vi "Frame Sync.vi"(6 "channel count (2)":u8=2, 7 "bit set edge (falling)":enum16{"rising", "falling"}(ring)=enum."falling", 9 "ready for input?":bool, 10 "transmit":bool, 11 "clock in":bool) -> (1 "ready for input":bool, 2 "latch config":bool, 3 "frame sync":bool)   [LabVIEW 2013, in "I2S-TDM.lvlib"]
uses:
  I2S-TDM.lvlib
  Controls/tdm transmit states.ctl
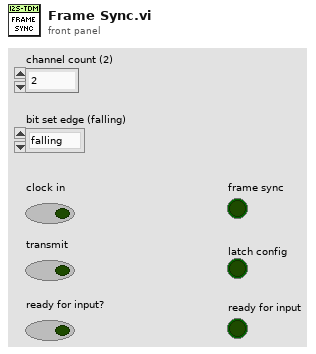
[diagram p1: front panel]
types:
  T1 = typedef "I2S-TDM.lvlib/tdm transmit states.ctl" = enum16{"idle", "pre-transfer", "transfer"}
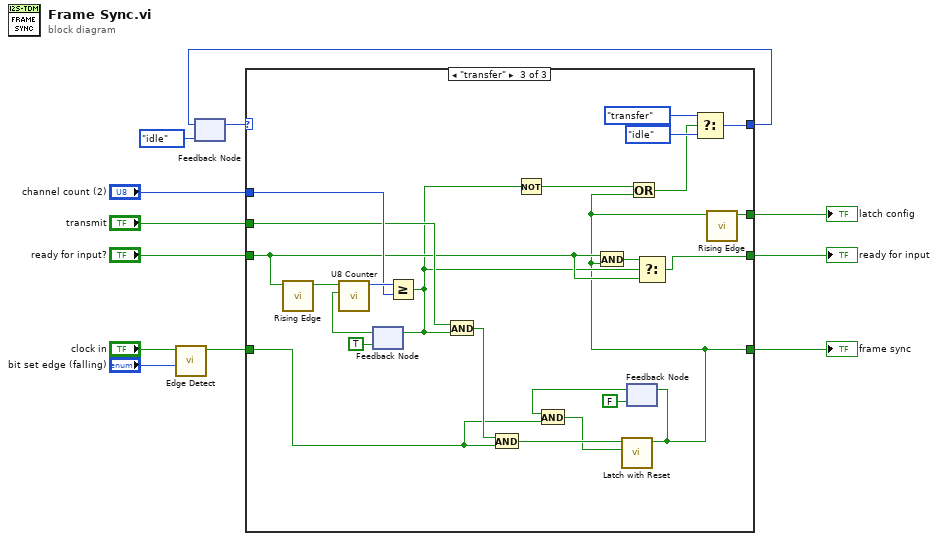
[diagram p0: block diagram]
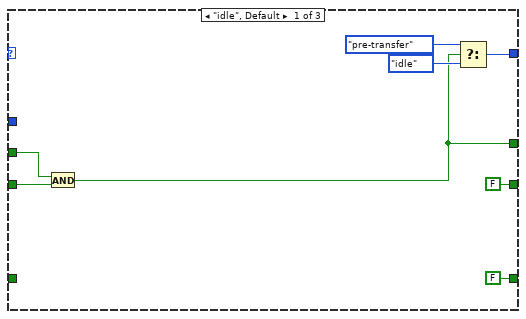
[diagram p2: hidden frame]
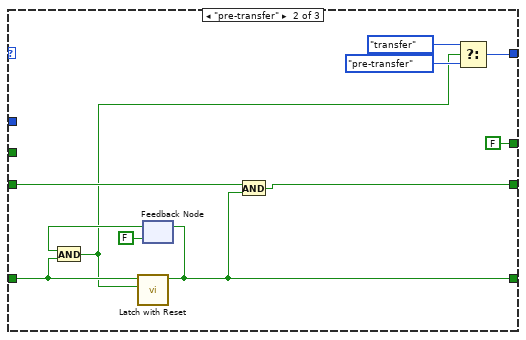
[diagram p3: hidden frame]
diagram:
  n1 = call "Edge Detect.vi"("edge (rising)"="bit set edge (falling)", "signal in"="clock in") -> ("edge detected?"=w6:bool)  [unwired: 9 in]
  n2 = feedback #1(tdm_transmit_states."idle") -> (w11:T1)
  n3 = case shown="\"transfer\"" w11 {
    tunnel: [w16 w26 w52] -> w10
    tunnel: "transmit" -> [w19 _ w48]
    tunnel: "ready for input?" -> [w20 w30 w42]
    tunnel: w6 -> [_ w25 w40]
    tunnel: [FALSE w29 w43] -> w5
    tunnel: [FALSE ("latched signal") w22 w32] -> w4
    tunnel: "channel count (2)" -> [_ _ w49]
    tunnel: [w13 FALSE w34] -> w2
    frame "idle", Default {
      n4 = And(x=w19, y=w20) -> (x .and. y?=w13:bool)
      n5 = Select(t=tdm_transmit_states."pre-transfer", s=w13, f=tdm_transmit_states."idle") -> (s? t:f=w16:T1)
    }
    frame "pre-transfer" {
      n6 = feedback #2(FALSE ("latched signal")) -> (w24:bool)
      n7 = And(x=w24, y=w25) -> (x .and. y?=w23:bool)
      n8 = call "Latch with Reset.vi"("reset"=w23, "signal"=w25) -> ("latched signal"=w22:bool)  [unwired: 9 in]
      n9 = feedback-in #2(w22) -> ()
      n10 = And(x=w30, y=w22) -> (x .and. y?=w29:bool)
      n11 = Select(t=tdm_transmit_states."transfer", s=w23, f=tdm_transmit_states."pre-transfer") -> (s? t:f=w26:T1)
    }
    frame "transfer" {
      n12 = call "Rising Edge.vi"("signal in"=w42) -> ("rising edge?"=w51:bool)  [unwired: 10 in]
      n13 = feedback #3(TRUE ("latched signal")) -> (w37:bool)
      n14 = call "U8 Counter.vi"("reset (F)"=w37, "increment"=w51) -> ("count"=w50:u8)  [unwired: 9 in]
      n15 = Greater Or Equal?(x=w50, y=w49) -> (x >= y?=w36:bool)
      n16 = feedback-in #3(w36) -> ()
      n17 = And(x=w48, y=w36) -> (x .and. y?=w44:bool)
      n18 = And(x=w44, y=w40) -> (x .and. y?=w46:bool)
      n19 = Not(x=w36) -> (.not. x?=w35:bool)
      n20 = feedback #4(FALSE ("latched signal")) -> (w45:bool)
      n21 = And(x=w45, y=w40) -> (x .and. y?=w39:bool)
      n22 = call "Latch with Reset.vi"("reset"=w39, "signal"=w46) -> ("latched signal"=w32:bool)  [unwired: 9 in]
      n23 = And(x=w42, y=w32) -> (x .and. y?=w41:bool)
      n24 = feedback-in #4(w32) -> ()
      n25 = Or(x=w35, y=w32) -> (x .or. y?=w33:bool)
      n26 = Select(t=w41, s=w36, f=w42) -> (s? t:f=w43:bool)
      n27 = Select(t=tdm_transmit_states."transfer", s=w33, f=tdm_transmit_states."idle") -> (s? t:f=w52:T1)
      n28 = call "Rising Edge.vi"("signal in"=w32) -> ("rising edge?"=w34:bool)  [unwired: 10 in]
    }
  }
  "ready for input" <- w5
  "frame sync" <- w4
  "latch config" <- w2
  n29 = feedback-in #1(w10) -> ()
